vi "is reference null.vi"(11 "reserver":T1 format="%.0x") -> (3 "Boolean":bool)   [LabVIEW 2016, in "FPGA RM System Definition API.lvlib"]
uses:
  <vilib>/NI Veristand/Custom Device API/Custom Device Item Ref.ctl
  FPGA-Resource-Manager-APIs/Source/System Definition/FPGA RM System Definition API.lvlib
  <vilib>/NI VeriStand/Custom Device API/Custom Device API.lvlib
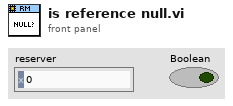
[diagram p1: front panel]
types:
  T1 = typedef "Custom Device API.lvlib/Custom Device Item Ref.ctl" = u64
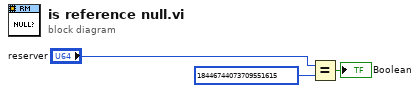
[diagram p0: block diagram]
diagram:
  n1 = Equal?(x="reserver", y=T1 18446744073709551615 ("reserver")) -> (x = y?=→"Boolean":bool)
